vi "Data to List.vi"(0 "Data String In":string, 11 "error in":errorcluster) -> (4 "Data List Out":refnum<k24>, 15 "error out":errorcluster)   [LabVIEW 2014, in "GEA2_Toolkit.lvlib"]
uses:
  library/GEA2_Toolkit.lvlib
panel:
  out "Data List Out 2":refnum<k24>
  out "error out 2":errorcluster
  in  "Data String In 2":string
  in  "error in 2":errorcluster
  out "Error Array 2":errorcluster[](array[cluster])
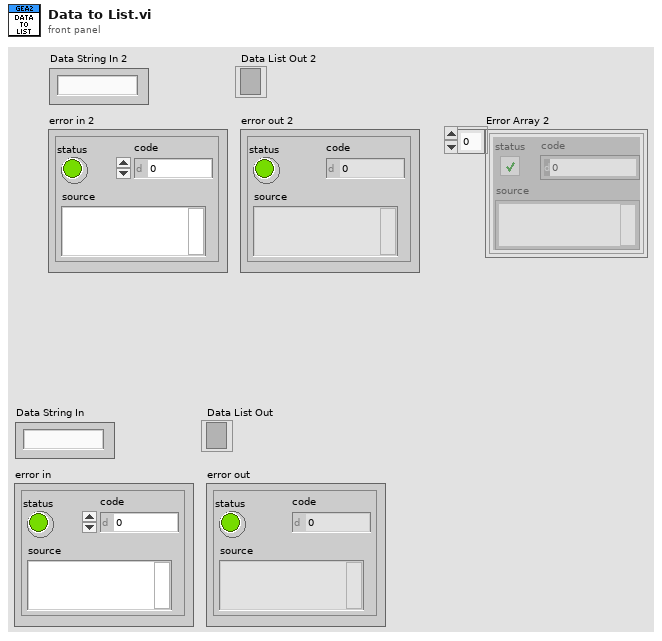
[diagram p1: front panel]
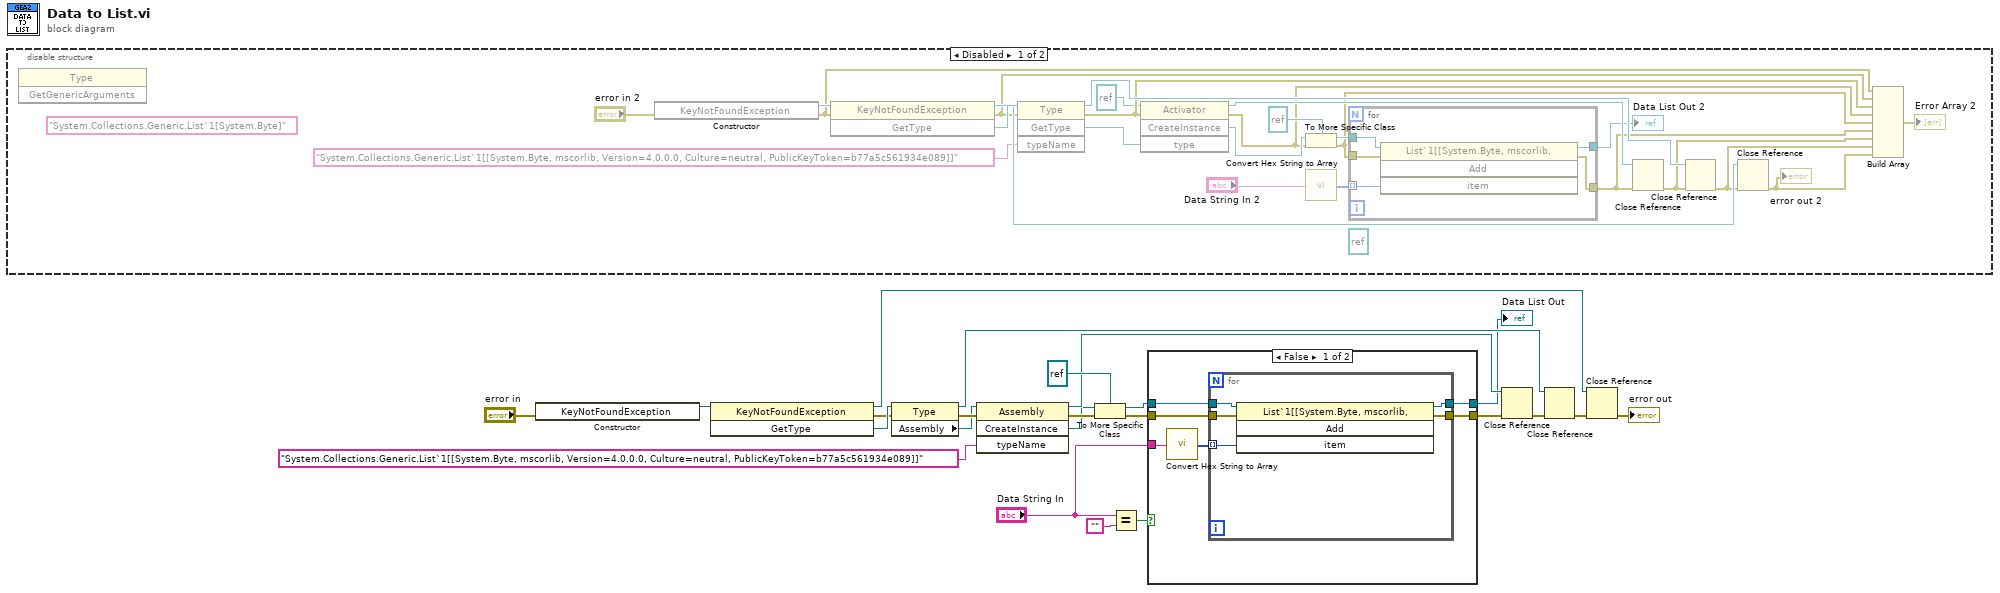
[diagram p0: block diagram]
diagram:
  n1 = disable-structure shown="Disabled" {
    frame Disabled {
      (unwired) "System.Collections.Generic.List`1[System.Byte]" ("typeName")
      (unwired) refnum<k24> refnum ("reference")
      n2 = invoke class="Type" method="GetGenericArguments"() -> ()  [unwired: 3 in, 3 out]
      n3 = constructor class="KeyNotFoundException"(error in="error in 2") -> (reference out=w41:refnum<k24>, error out=w37:errorcluster)  [unwired: 2 in, 1 out]
      n4 = invoke class="KeyNotFoundException" method="GetType"(reference=w41, error in=w37) -> (reference out=w47:refnum<k24>, error out=w35:errorcluster, "GetType"=w48:refnum<k24>)  [unwired: 1 in]
      n5 = invoke class="Type" method="GetType"(reference=w48, error in=w35, "typeName"="System.Collections.Generic.List`1[[System.Byte, mscorlib, Version=4.0.0.0, Culture=neutral, PublicKeyToken=b77a5c561934e089]]") -> (reference out=w40:refnum<k24>, error out=w32:errorcluster, "GetType"=w46:refnum<k24>)  [unwired: 1 in, 1 out]
      n6 = invoke class="Activator" method="CreateInstance"(reference=refnum<k24> refnum, error in=w32, "type"=w46) -> (reference out=w45:refnum<k24>, error out=w27:errorcluster, "CreateInstance"=w42:refnum<k24>)  [unwired: 1 in, 1 out]
      n7 = To More Specific Class(target class=refnum<k24> refnum ("reference"), reference=w42, error in=w27) -> (specific class reference=w43:refnum<k24>, error out=w28:errorcluster)
      n8 = call "Convert Hex String to Array.vi"("Hex String In"="Data String In 2") -> ("Hex Array Out"=w26:u8[])  [unwired: 14 in]
      n9 = for {
        tunnel: w26 -> [w52] mode=indexing
        tunnel: w28 -> [w50]
        tunnel: [w51] -> w29
        tunnel: w43 -> [w49]
        tunnel: [w53] -> w24
        n10 = invoke class="List`1[[System.Byte, mscorlib, " method="Add"(reference=w49, error in=w50, "item"=w52) -> (reference out=w53:refnum<k24>, error out=w51:errorcluster)  [unwired: 1 in, 2 out]
      }
      "Data List Out 2" <- w24
      n11 = Close Reference(reference=w45, error in (no error)=w29) -> (error out=w33:errorcluster)
      n12 = Close Reference(reference=w40, error in (no error)=w33) -> (error out=w38:errorcluster)
      n13 = Close Reference(reference=w47, error in (no error)=w38) -> (error out=w39:errorcluster)
      "error out 2" <- w39
      n14 = Build Array(w37, w35, w32, w27, w28, w29, w33, w38, w39) -> (→"Error Array 2":errorcluster[])
    }
    frame Enabled {
    }
  }
  n15 = constructor class="KeyNotFoundException"(error in="error in") -> (reference out=w18:refnum<k24>)  [unwired: 2 in, 2 out]
  n16 = invoke class="KeyNotFoundException" method="GetType"(reference=w18) -> (reference out=w16:refnum<k24>, error out=w14:errorcluster, "GetType"=w15:refnum<k24>)  [unwired: 2 in]
  n17 = property class="Type"(reference=w15, error in=w14) -> (reference out=w13:refnum<k24>, error out=w8:errorcluster, "Assembly"=w6:refnum<k24>)
  n18 = invoke class="Assembly" method="CreateInstance"(reference=w6, error in=w8, "typeName"="System.Collections.Generic.List`1[[System.Byte, mscorlib, Version=4.0.0.0, Culture=neutral, PublicKeyToken=b77a5c561934e089]]") -> (reference out=w9:refnum<k24>, error out=w10:errorcluster, "CreateInstance"=w4:refnum<k24>)  [unwired: 1 in, 1 out]
  n19 = To More Specific Class(target class=refnum<k24> refnum ("reference"), reference=w4, error in=w10) -> (specific class reference=w7:refnum<k24>, error out=w22:errorcluster)
  n20 = Equal?(x="Data String In", y="") -> (x = y?=w2:bool)
  n21 = case shown="False" w2 {
    tunnel: [w59 w66] -> w1
    tunnel: w22 -> [w57 w65]
    tunnel: [w56 w65] -> w12
    tunnel: w7 -> [w55 w66]
    tunnel: "Data String In" -> [w54 _]
    frame False {
      n22 = call "Convert Hex String to Array.vi"("Hex String In"=w54) -> ("Hex Array Out"=w58:u8[])  [unwired: 14 in]
      n23 = for {
        tunnel: w58 -> [w63] mode=indexing
        tunnel: w57 -> [w61]
        tunnel: [w62] -> w56
        tunnel: w55 -> [w60]
        tunnel: [w64] -> w59
        n24 = invoke class="List`1[[System.Byte, mscorlib, " method="Add"(reference=w60, error in=w61, "item"=w63) -> (reference out=w64:refnum<k24>, error out=w62:errorcluster)  [unwired: 1 in, 2 out]
      }
    }
    frame True {
    }
  }
  "Data List Out" <- w1
  n25 = Close Reference(reference=w9, error in (no error)=w12) -> (error out=w5:errorcluster)
  n26 = Close Reference(reference=w13, error in (no error)=w5) -> (error out=w20:errorcluster)
  n27 = Close Reference(reference=w16, error in (no error)=w20) -> (error out=→"error out":errorcluster)
